vi "Daqmx_DigOut.vi"(3 "error in":errorcluster, 4 "Array of Ports, Lines":u8[][](array[numeric]), 5 "Base Task Name":string, 6 "DAQmx device name":string) -> (0 "error out":errorcluster, 2 "Output Task Name":refnum<k21>)   [LabVIEW 2014]
uses:
  <vilib>/DAQmx/create/channels.llb/DAQmx Create Channel (DO-Digital Output).vi
panel:
  out "Channel List":string
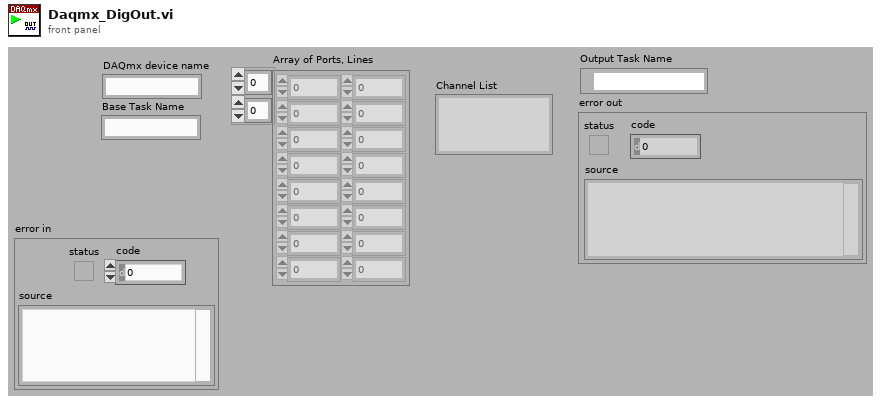
[diagram p1: front panel]
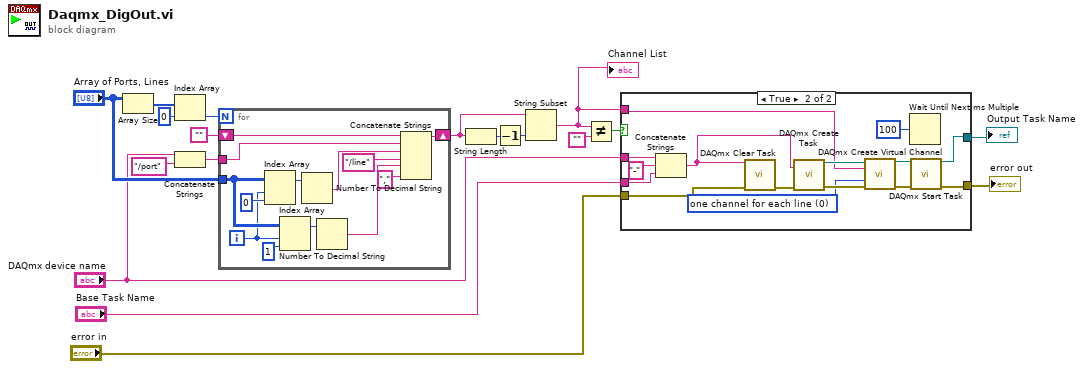
[diagram p0: block diagram]
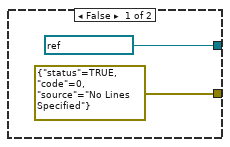
[diagram p2: hidden frame]
diagram:
  n1 = Array Size(array="Array of Ports, Lines") -> (size(s)=w16:i32[])
  n2 = Index Array(array=w16, index=0) -> (element=w15:i32)
  n3 = Concatenate Strings("DAQmx device name", "/port" ("string")) -> (w12:string)
  n4 = for {
    N: w15 -> [_]
    shift-right: [w31] -> w10
    shift-left: "" -> [w30]
    tunnel: w12 -> [w26]
    tunnel: "Array of Ports, Lines" -> [w24]
    i -> [w19]
    n5 = Index Array(array=w24, index (row)=w19, index (col)=0 ("disabled index (col)")) -> (element=w29:u8)
    n6 = Index Array(array=w24, index (row)=w19, index (col)=1 ("disabled index (col)")) -> (element=w25:u8)
    n7 = Number To Decimal String(number=w29) -> (decimal integer string=w28:string)  [unwired: 1 in]
    n8 = Number To Decimal String(number=w25) -> (decimal integer string=w23:string)  [unwired: 1 in]
    n9 = Concatenate Strings(w30, w26, w28, "/line" ("string"), w23, "," ("string")) -> (w31:string)
  }
  n10 = String Length(string=w10) -> (length=w11:i32)
  n11 = Decrement(x=w11) -> (x-1=w9:i32)
  n12 = String Subset(string=w10, length (rest)=w9) -> (substring=w1:string)  [unwired: 1 in]
  "Channel List" <- w1
  n13 = Not Equal?(x=w1, y="") -> (x != y?=w6:bool)
  n14 = case shown="True" w6 {
    tunnel: "Base Task Name" -> [_ w42]
    tunnel: "DAQmx device name" -> [_ w41]
    tunnel: w1 -> [_ w40]
    tunnel: [errorcluster {"status"=TRUE, "code"=0, "source"="No Lines Specified"} ("error out") w39] -> w4
    tunnel: [refnum<k21> "Empty Task" ("task out") w34] -> w3
    tunnel: "error in" -> [_ w37]
    frame False {
    }
    frame True {
      w44 = 0 items=["one channel for each line", "one channel for all lines"] ("line grouping")
      n15 = Concatenate Strings(w41, "-" ("new task name"), w42) -> (w36:string)
      n16 = call <vilib>:"DAQmx Clear Task.vi"("task in"=w36, "error in"=w37) -> ("error out"=w35:errorcluster)  [unwired: 13 in]
      n17 = call <vilib>:"DAQmx Create Task.vi"("new task name"=w36, "error in"=w35) -> ("task out"=w47:refnum<k21>, "error out"=w46:errorcluster)  [unwired: 12 in]
      n18 = call-poly <vilib>:"DAQmx Create Virtual Channel.vi"("task in"=w47, "lines"=w40, "line grouping"=w44, "error in"=w46) -> ("task out"=w43:refnum<k21>, "error out"=w45:errorcluster)  [unwired: 10 in]
      n19 = Wait Until Next ms Multiple(millisecond multiple=u32 100) -> ()  [unwired: 1 out]
      n20 = call <vilib>:"DAQmx Start Task.vi"("task/channels in"=w43, "error in"=w45) -> ("task out"=w34:refnum<k21>, "error out"=w39:errorcluster)  [unwired: 12 in]
    }
  }
  "error out" <- w4
  "Output Task Name" <- w3
